vi "Get_AI.vi"(8 "error in (no error)":errorcluster, 10 "PIN Number":i8, 11 "Driver_AI_AO in":refnum<class "Driver_AI_AO.lvclass">) -> (0 "error out":errorcluster, 2 "STATUS":string, 3 "Driver_AI_AO out":refnum<class "Driver_AI_AO.lvclass">)   [LabVIEW 2023, in "Driver_AI_AO.lvlib" / "Driver_AI_AO.lvclass"]
uses:
  Driver_AI_AO.lvclass
  Driver_AI_AO.lvclass/Driver_AI_AO.ctl
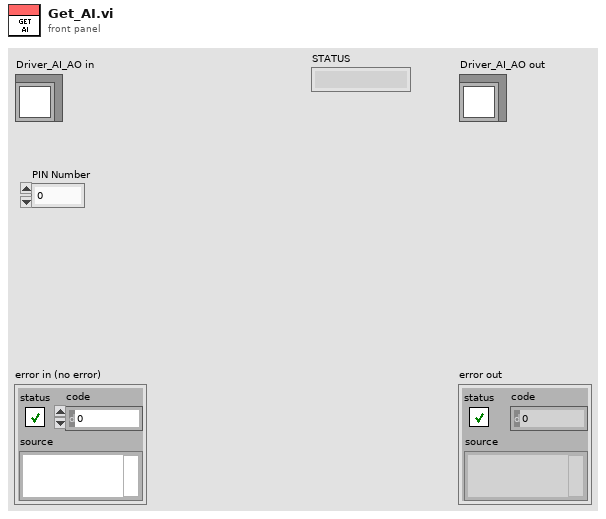
[diagram p1: front panel]
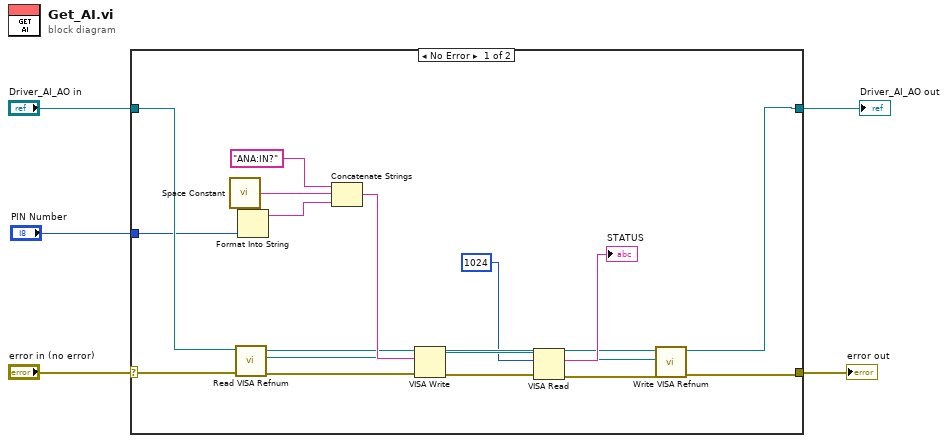
[diagram p0: block diagram]
diagram:
  n1 = case shown="No Error" "error in (no error)" {
    selector: "error in (no error)" -> [w10 w25]
    tunnel: [w9 w25] -> w4
    tunnel: [w7 w24] -> w2
    tunnel: "Driver_AI_AO in" -> [w8 w24]
    tunnel: "PIN Number" -> [w6 _]
    frame No Error {
      n2 = call <vilib>:"Space Constant.vi"() -> ("String"=w21:string)
      n3 = call-dynamic "Read VISA Refnum.vi"("error in (no error)"=w10, "Driver in"=w8) -> ("error out"=w16:errorcluster, "VISA Refnum"=w15:refnum<visa-resource-name>, "Driver out"=w18:refnum<class "Driver_AI_AO.lvclass">)  [unwired: 7 in]
      n4 = Format Into String(w6) -> (resulting string=w22:string)  [unwired: 3 in, 1 out]
      n5 = Concatenate Strings("ANA:IN?" ("string"), w21, w22) -> (w23:string)
      n6 = VISA Write(VISA resource name=w15, write buffer=w23, error in (no error)=w16) -> (VISA resource name out=w14:refnum<visa-resource-name>, error out=w13:errorcluster)  [unwired: 1 out]
      n7 = VISA Read(VISA resource name=w14, byte count=u32 1024, error in (no error)=w13) -> (VISA resource name out=w19:refnum<visa-resource-name>, read buffer=→"STATUS":string, error out=w17:errorcluster)  [unwired: 1 out]
      n8 = call-dynamic "Write VISA Refnum.vi"("error in (no error)"=w17, "VISA Refnum"=w19, "Driver in"=w18) -> ("error out"=w9:errorcluster, "Driver out"=w7:refnum<class "Driver_AI_AO.lvclass">)  [unwired: 7 in]
    }
    frame Error {
    }
  }
  "error out" <- w4
  "Driver_AI_AO out" <- w2
